vi "Access Many Float.vi"(6 "Defaults":dbl[](array[numeric]), 7 "Get/Set":enum16{"Get", "Set"}(ring), 8 "error in (no error)":errorcluster, 9 "Values in":dbl[](array[numeric]), 10 "Keys":string[](array[string]), 11 "FlexWorktable in":refnum<class "FlexWorktable.lvclass">) -> (0 "error out":errorcluster, 2 "Values out":dbl[](array[numeric]), 3 "FlexWorktable out":refnum<class "FlexWorktable.lvclass">)   [LabVIEW 2023, in "FlexWorktable.lvclass"]
uses:
  FlexWorktable.lvclass
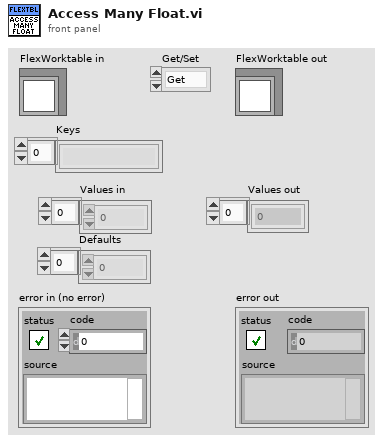
[diagram p1: front panel]
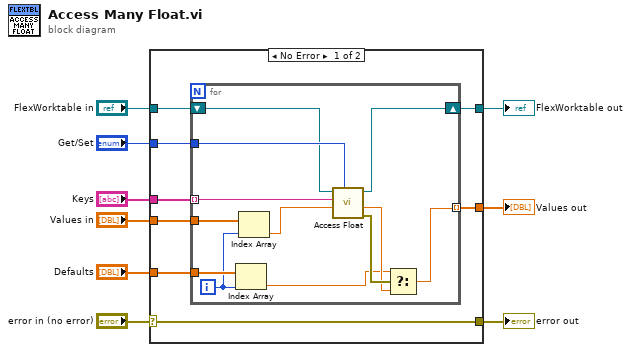
[diagram p0: block diagram]
diagram:
  n1 = case shown="No Error" "error in (no error)" {
    selector: "error in (no error)" -> [w10 w31]
    tunnel: [w10 w31] -> w8
    tunnel: [w12 w30] -> w6
    tunnel: "FlexWorktable in" -> [w16 w30]
    tunnel: "Keys" -> [w17 _]
    tunnel: "Get/Set" -> [w15 _]
    tunnel: "Values in" -> [w14 _]
    tunnel: [w13 _] -> w2
    tunnel: "Defaults" -> [w11 _]
    frame No Error {
      n2 = for {
        tunnel: w17 -> [w29] mode=indexing
        tunnel: w15 -> [w28]
        shift-right: [w26] -> w12
        shift-left: w16 -> [w27]
        tunnel: w14 -> [w21]
        tunnel: [w23] -> w13 mode=indexing
        tunnel: w11 -> [w22]
        i -> [w20]
        n3 = Index Array(array=w22, index=w20) -> (element=w18:dbl)
        n4 = Index Array(array=w21, index=w20) -> (element=w19:dbl)
        n5 = call-dynamic "Access Float.vi"("Get/Set"=w28, "Value in"=w19, "Key"=w29, "FlexWorktable in"=w27) -> ("error out"=w25:errorcluster, "Value out"=w24:dbl, "FlexWorktable out"=w26:refnum<class "FlexWorktable.lvclass">)  [unwired: 5 in]
        n6 = Select(t=w18, s=w25, f=w24) -> (s? t:f=w23:dbl)
      }
    }
    frame Error {
    }
  }
  "error out" <- w8
  "FlexWorktable out" <- w6
  "Values out" <- w2
